vi "MB Slave Read Discrete Inputs (poly).vi"(1 "Starting Address":u16, 2 "Quantity":u16, 5 "error in":errorcluster) -> (15 "Discrete Inputs":bool[](array[boolean]), 19 "error out":errorcluster)   [LabVIEW 2023, in "Voegtlin_NI_SMART_Modbus_Drivers.lvlib"]
doc: "Returns the slave's discrete inputs from Starting Address to Starting Address + Quantity."
uses:
  Voegtlin_NI_SMART_Modbus_Drivers.lvlib
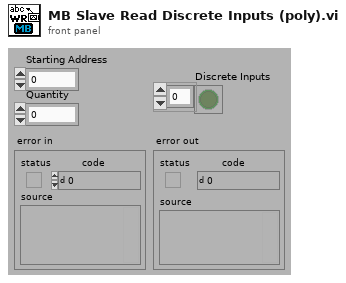
[diagram p1: front panel]
types:
  T1 = enum16{"Discrete Inputs", "Coils", "Input Registers", "Holding Registers"}
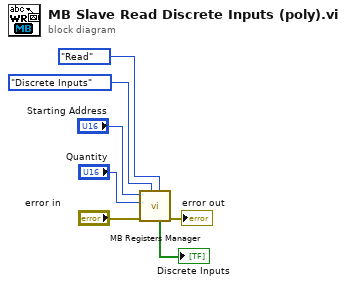
[diagram p0: block diagram]
diagram:
  n1 = call "MB Registers Manager.vi"("Function"=enum16{"Init", "Read", "Write", "Read All"}."Read", "Table"=T1."Discrete Inputs", "error in (no error)"="error in", "Length"="Quantity", "Start Address"="Starting Address") -> ("error out"=→"error out":errorcluster, "Bits out"=→"Discrete Inputs":bool[])  [unwired: 2 in, 3 out]
